vi "DICOMServerSettings.vi"() -> ()   [LabVIEW 2013, in "main.lvlib"]
uses:
  main.lvlib
  Controls/Enum Save Action Events.ctl
  Controls/SaveDataCluster.ctl
  <vilib>/Utility/cursorutil.llb/Set Cursor (Icon Pict).vi
panel:
  out "QueryRequestStr":string="Edit query request"
  in  "Cancel":bool
  in  "Save":bool
  in  "Port PACS":i32 caption="Port"
  in  "Host PACS":string caption="Host"
  in  "Remote AE Title PACS":string caption="Remote AE Title"
  in  "Client AE Title PACS":string caption="Client AE Title"
  in  "Port":i32
  in  "Host":string
  in  "Remote AE Title":string
  in  "Client AE Title":string
  # "Worklist Server Details"
  # "PACS Server Details"
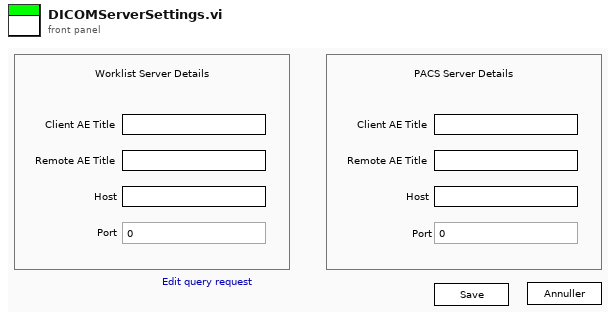
[diagram p1: front panel]
types:
  T1 = typedef "main.lvlib/SaveDataCluster.ctl" = cluster{"HospInfo":cluster{"Name":string, "Address":string, "Department":string}, "Pressure":cluster{"Pressure":dbl}, "DataPath":cluster{"DataPath":path}, "ReportPath":cluster{"Path":path, "Name":string}, "DICOM Info WL":cluster{"port":i32, "AEtitle":string, "host":string, "remoteAE":string}, "DICOM Info PACS":cluster{"port":i32, "AEtitle":string, "host":string, "remoteAE":string}, "ArmCalcMethod":dbl, "itemTags":string[], "DicomEncoding":u16, "JournalType":u16, "General Settings":cluster{"Hyphenation":bool, "Language":u16, "CellStr1":string, "CellStr2":string}, "Dicom Tags":string[][], "BT Serial":cluster{"Serial Number":string, "Side":string, "Ignore?":bool}[], "BT License":cluster{"License":string, "Accepted Serials":string[]}}
  T2 = typedef "main.lvlib/Enum Save Action Events.ctl" = enum16{"LoadReportPath", "SaveReportPath", "Load Graph Path", "Save Graph Path", "LoadDataPath", "SaveDataPath", "Load Template Path", "Save Template Path", "Load PressureFactor", "Save PressureFactor", "Init", "Load Listbox", "Save Listbox", "LoadHospInfo", "SaveHospInfo", "Load DICOM Activation", "Save DICOM Activation", "LoadDICOMInfoWL", "SaveDICOMInfoWL", "LoadDICOMInfoPACS", "SaveDICOMInfoPACS", "Load ArmCalcMethod", "Save ArmCalcMethod", "LoadItemTags", "SaveItemTags", "LoadDICOMEncoding", "SaveDICOMEncoding", "LoadJournalType", "SaveJournalType", "LoadAcqFilterType", "SaveAcqFilterType", "Load Sequence", "Save Sequence", "Load Acquisition Mode", "Save Acquisition Mode", "Load General Settings", "Save General Settings", "Load Language", "Save Language", "Load Dicom Tags", "Save Dicom Tags", "Load BT Serial", "Save BT Serial", "Load BT License", "Save BT License"}
  T3 = cluster{"port":i32, "AEtitle":string, "host":string, "remoteAE":string}
  T4 = cluster{"Port":i32, "Client AE Title":string, "Host":string, "Remote AE Title":string}
  T5 = cluster{"Port PACS":i32, "Client AE Title PACS":string, "Host PACS":string, "Remote AE Title PACS":string}
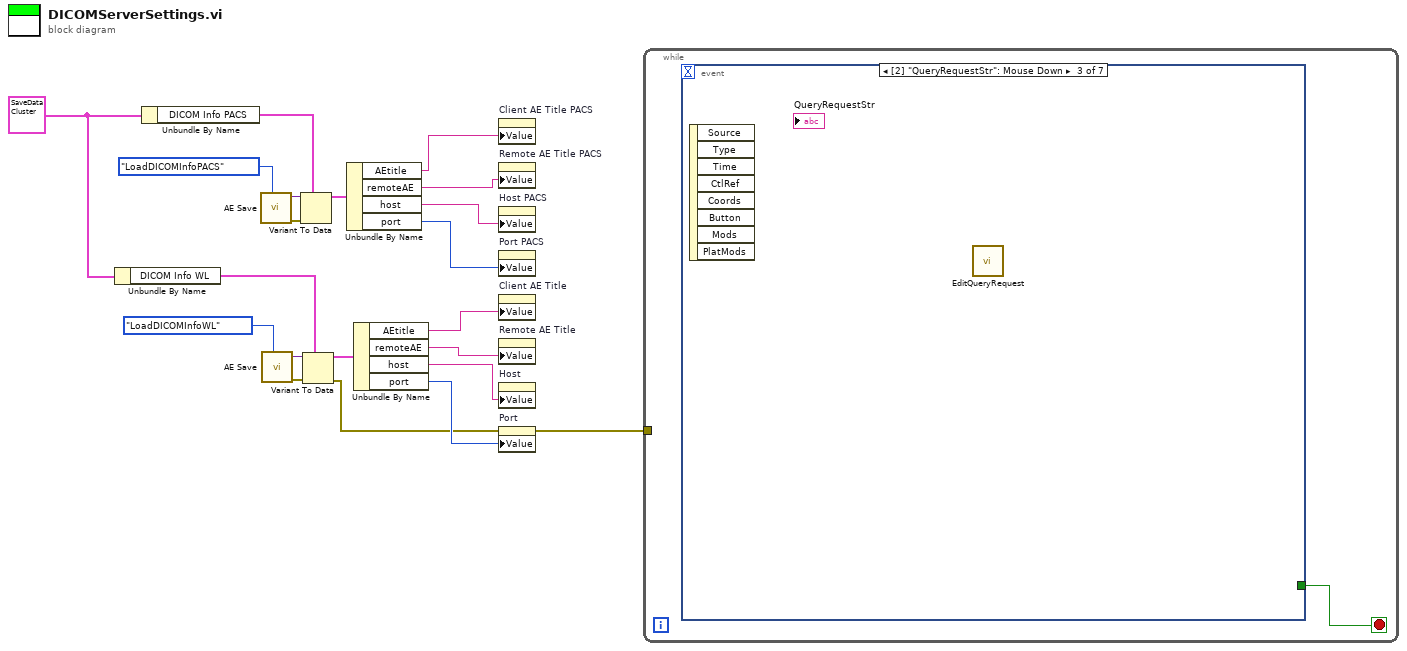
[diagram p0: block diagram]
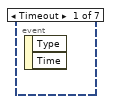
[diagram p2: hidden frame]
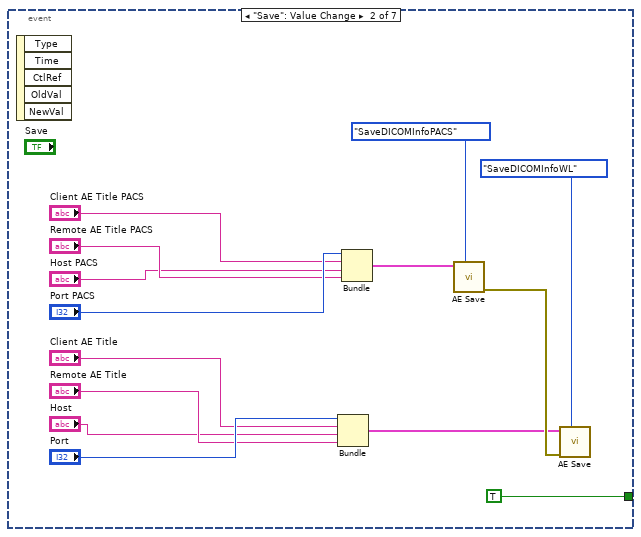
[diagram p3: hidden frame]
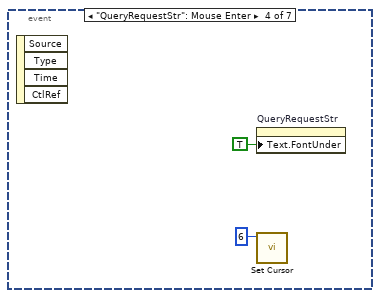
[diagram p4: hidden frame]
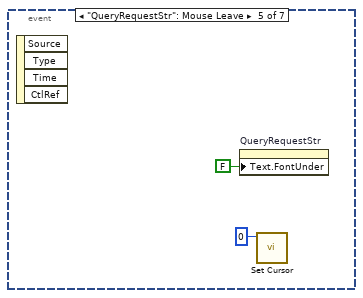
[diagram p5: hidden frame]
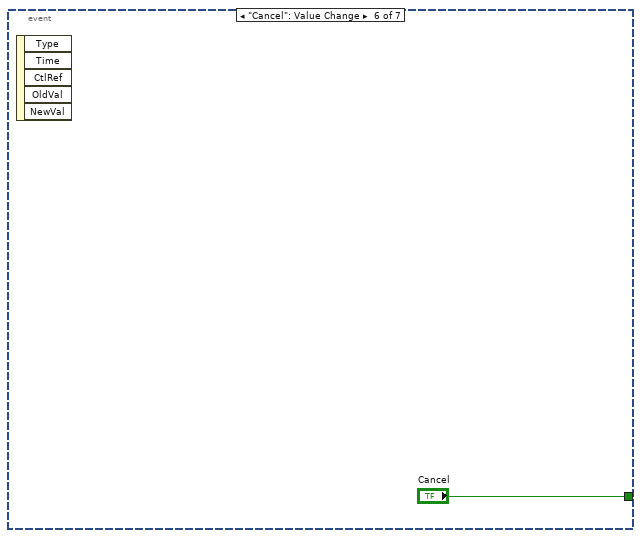
[diagram p6: hidden frame]
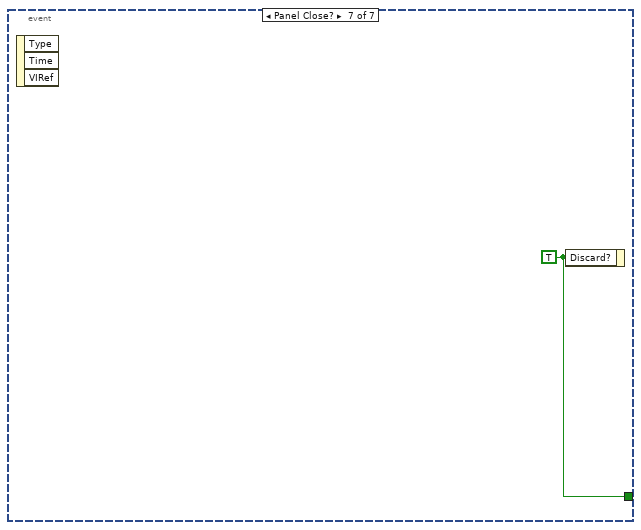
[diagram p7: hidden frame]
diagram:
  w1 = T1 {"HospInfo"={"Name"="", "Address"="", "Department"=""}, "Pressure"={"Pressure"=0.0}, "DataPath"={"DataPath"=path ""}, "ReportPath"={"Path"=path "", "Name"=""}, "DICOM Info WL"={"port"=0, "AEtitle"="", "host"="", "remoteAE"=""}, "DICOM Info PACS"={"port"=0, "AEtitle"="", "host"="", "remoteAE"=""}, "ArmCalcMethod"=0.0, "itemTags"=[], "DicomEncoding"=0, "JournalType"=0, "General Settings"={"Hyphenation"=FALSE, "Language"=0, "CellStr1"="", "CellStr2"=""}, "Dicom Tags"=[], "BT Serial"=[], "BT License"={"License"="", "Accepted Serials"=[]}} ("Data")
  n1 = Unbundle By Name(w1) -> ("DICOM Info WL"=w14:T3)
  n2 = Unbundle By Name(w1) -> ("DICOM Info PACS"=w17:T3)
  n3 = call "AE Save.vi"("Action"=Enum_Save_Action_Events."LoadDICOMInfoPACS") -> ("error out"=w19:errorcluster, "Anything"=w18:variant)  [unwired: 8 in]
  n4 = call "AE Save.vi"("Action"=Enum_Save_Action_Events."LoadDICOMInfoWL") -> ("error out"=w15:errorcluster, "Anything"=w16:variant)  [unwired: 8 in]
  n5 = Variant To Data(error in=w19, type=w17, Variant=w18) -> (data=w12:T3)  [unwired: 1 out]
  n6 = Variant To Data(error in=w15, type=w14, Variant=w16) -> (data=w13:T3, error out=w2:errorcluster)
  n7 = Unbundle By Name(w12) -> ("AEtitle"=w11:string, "remoteAE"=w10:string, "host"=w9:string, "port"=w8:i32)
  n8 = Unbundle By Name(w13) -> ("AEtitle"=w4:string, "remoteAE"=w5:string, "host"=w6:string, "port"=w7:i32)
  n9 = property on="Client AE Title PACS" class="Str"("Value"=w11) -> ()  [unwired: 2 in, 2 out]
  n10 = property on="Remote AE Title PACS" class="Str"("Value"=w10) -> ()  [unwired: 2 in, 2 out]
  n11 = property on="Host PACS" class="Str"("Value"=w9) -> ()  [unwired: 2 in, 2 out]
  n12 = property on="Port PACS" class="DigNum (strict)"("Value"=w8) -> ()  [unwired: 2 in, 2 out]
  n13 = property on="Client AE Title" class="Str"("Value"=w4) -> ()  [unwired: 2 in, 2 out]
  n14 = property on="Remote AE Title" class="Str"("Value"=w5) -> ()  [unwired: 2 in, 2 out]
  n15 = property on="Host" class="Str"("Value"=w6) -> ()  [unwired: 2 in, 2 out]
  n16 = property on="Port" class="DigNum (strict)"(error in=w2, "Value"=w7) -> (error out=w3:errorcluster)  [unwired: 1 in, 1 out]
  n17 = while {
    tunnel: w3 -> [_]
    stop <- w22 stop-if-true
    n18 = event shown="[2] \"QueryRequestStr\": Mouse Down" {
      selector: _ -> [_ _ _ _ _ _ _]
      dyn-events: _ -> [_ _ _ _ _ _ _]
      timeout: _ -> [_ _ _ _ _ _ _]
      tunnel: [_ TRUE _ _ _ "Cancel" w42] -> w22
      event Timeout {
        n19 = event-data() -> ()  [unwired: 1 in, 2 out]
      }
      event "Save": Value Change {
        n20 = event-data() -> ()  [unwired: 1 in, 5 out]
        n21 = Bundle("Port"="Port", "Client AE Title"="Client AE Title", "Host"="Host", "Remote AE Title"="Remote AE Title") -> (w34:T4)  [unwired: 1 in]
        n22 = Bundle("Port PACS"="Port PACS", "Client AE Title PACS"="Client AE Title PACS", "Host PACS"="Host PACS", "Remote AE Title PACS"="Remote AE Title PACS") -> (w25:T5)  [unwired: 1 in]
        n23 = call "AE Save.vi"("Variant In"=w25, "Action"=Enum_Save_Action_Events."SaveDICOMInfoPACS") -> ("error out"=w35:errorcluster)  [unwired: 7 in, 1 out]
        n24 = call "AE Save.vi"("error in (no error)"=w35, "Variant In"=w34, "Action"=Enum_Save_Action_Events."SaveDICOMInfoWL") -> ()  [unwired: 6 in, 2 out]
      }
      event "QueryRequestStr": Mouse Down {
        n25 = event-data() -> ()  [unwired: 1 in, 8 out]
        n26 = call "EditQueryRequest.vi"() -> ()  [unwired: 11 in, 1 out]
      }
      event "QueryRequestStr": Mouse Enter {
        n27 = event-data() -> ()  [unwired: 1 in, 4 out]
        n28 = property on="QueryRequestStr" class="Str"("Text.FontUnder"=TRUE ("Text.Font:Underline")) -> ()  [unwired: 2 in, 2 out]
        n29 = call-poly <vilib>:"Set Cursor.vi"("icon"=u16 6) -> ()  [unwired: 9 in, 2 out]
      }
      event "QueryRequestStr": Mouse Leave {
        n30 = event-data() -> ()  [unwired: 1 in, 4 out]
        n31 = property on="QueryRequestStr" class="Str"("Text.FontUnder"=FALSE ("Text.Font:Underline")) -> ()  [unwired: 2 in, 2 out]
        n32 = call-poly <vilib>:"Set Cursor.vi"("icon"=u16 0) -> ()  [unwired: 9 in, 2 out]
      }
      event "Cancel": Value Change {
        n33 = event-data() -> ()  [unwired: 1 in, 5 out]
      }
      event Panel Close? {
        w42 = TRUE ("Discard?")
        n34 = event-data() -> ()  [unwired: 1 in, 3 out]
        n35 = event-data("Discard?"=w42) -> ()  [unwired: 1 in, 1 out]
      }
    }
  }
